vi "Enable.vi"   [LabVIEW 2018, in "Aerotech.lvlib"]
uses:
  Aerotech.lvlib
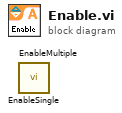
[diagram p0: block diagram]
diagram:
  n1 = call "EnableSingle.vi"() -> ()  [unwired: 10 in, 2 out]
  n2 = call "EnableMultiple.vi"() -> ()  [unwired: 10 in, 2 out]
